vi "Write effective exptime.vi"(8 "error in (no error)":errorcluster, 10 "effective exptime":dbl, 11 "Simulated Camera in":refnum<class "Simulated Camera.lvclass">) -> (0 "error out":errorcluster, 3 "Simulated Camera out":refnum<class "Simulated Camera.lvclass">)   [LabVIEW 2018, in "Simulated Camera.lvclass"]
uses:
  Simulated Camera.lvclass
  Simulated Camera.lvclass/Simulated Camera.ctl
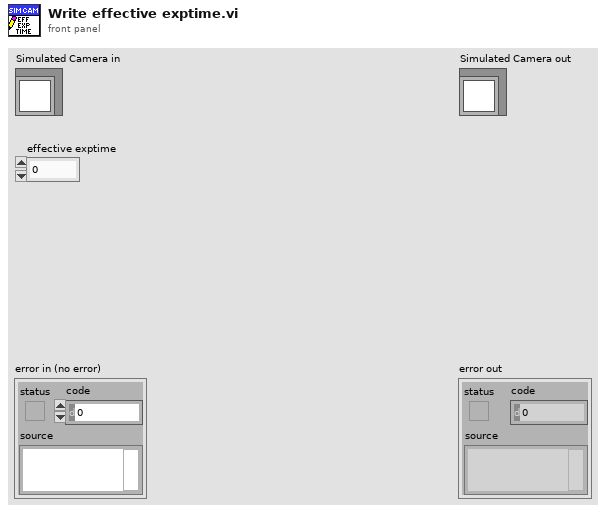
[diagram p1: front panel]
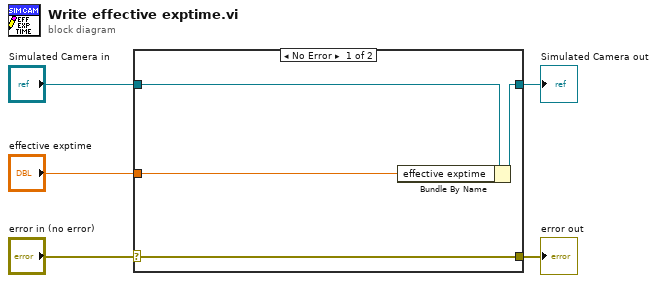
[diagram p0: block diagram]
diagram:
  n1 = case shown="No Error" "error in (no error)" {
    selector: "error in (no error)" -> [w9 w10]
    tunnel: [w9 w10] -> w4
    tunnel: [w7 w11] -> w2
    tunnel: "Simulated Camera in" -> [w8 w11]
    tunnel: "effective exptime" -> [w6 _]
    frame No Error {
      n2 = Bundle By Name(cluster=w8, "effective exptime"=w6) -> (w7:refnum<class "Simulated Camera.lvclass">)
    }
    frame Error {
    }
  }
  "error out" <- w4
  "Simulated Camera out" <- w2
